vi "模拟输入_连续(IEPE_频域).vi"() -> ()   [LabVIEW 2013]
doc: "This example demonstrates how to acquire a continuous data."
uses:
  <userlib>/ArtDAQ/_SubVI/ArtDAQ_CreateAIVoltageIEPEChan.vi
  <userlib>/ArtDAQ/_SubVI/ArtDAQ_CfgSampClkTiming.vi
  <userlib>/ArtDAQ/_SubVI/ArtDAQ_CfgDigEdgeStartTrig.vi
  <userlib>/ArtDAQ/_SubVI/ArtDAQ_CfgAnlgEdgeStartTrig.vi
  <userlib>/ArtDAQ/_SubVI/ArtDAQ_Read Analog DBL NChan NSamp.vi
  <vilib>/measure/maspectr.llb/FFT Power Spectrum and PSD for 1 Chan.vi
  <vilib>/measure/NI_MAPro.lvlib
panel:
  out "波形图":cluster{"f0":dbl, "df":dbl, "magnitude":dbl[]}[](graph)
  in  "耦合":i32(ring)=10050 items=["交流耦合"=10045, "直流耦合"=10050, "接地"=10066]
  in  "触发模式":enum32{"无触发", "数字边沿", "模拟边沿"}(tab)
  in  "触发源":string="/Dev1/PFI1"
  in  "触发边沿":i32(ring)=10280 items=["上升"=10280, "下降"=10171]
  in  "触发电平(V)":dbl
  in  "触发源":string(combo)="Dev1/ai0"
  in  "斜率":i32(ring)=10280 items=["上升"=10280, "下降"=10171]
  in  "停止":bool
  out "波形图":dbl[][](graph)
  in  "采样速率":dbl=10000.0 format="%#_13g"
  in  "每通道采样数":i32=1000
  in  "接线端配置":i32(ring)=12529 items=["默认"=-1, "单端"=10083, "非参考单端"=10078, "差分"=10106, "伪差分"=12529]
  in  "最小值(V)":dbl=-11.0 format="%#_13g"
  in  "最大值(V)":dbl=11.0 format="%#_13g"
  in  "物理通道":string(combo)="Dev1/ai0"
  out "错误":errorcluster
  # "通道属性"
  # "定时"
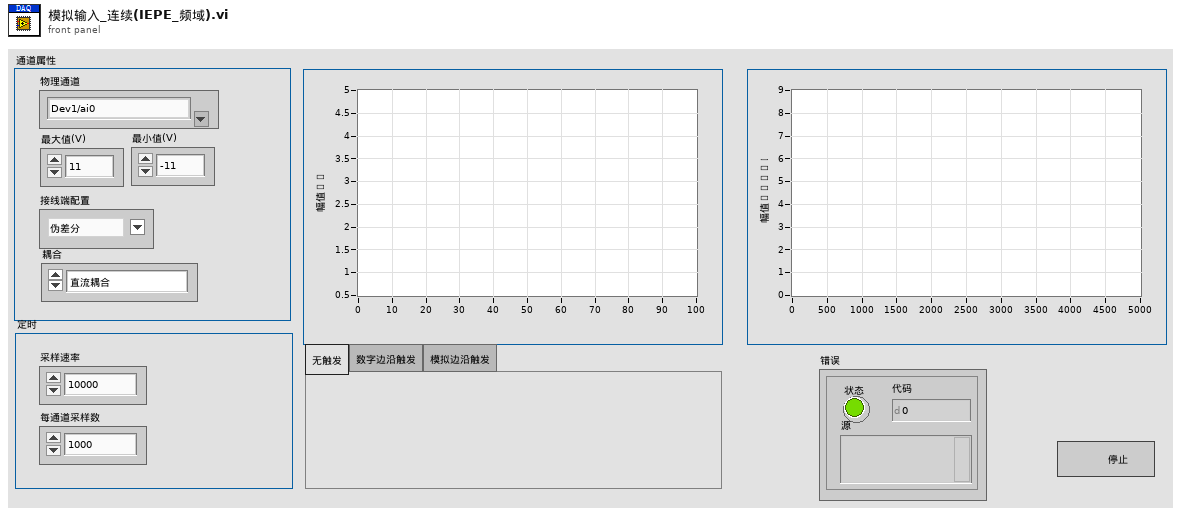
[diagram p1: front panel]
types:
  T1 = cluster{"averaging mode":enum16{"No averaging", "Vector averaging", "RMS averaging", "Peak hold"}, "weighting mode":enum16{"Linear", "Exponential"}, "number of averages":u32}
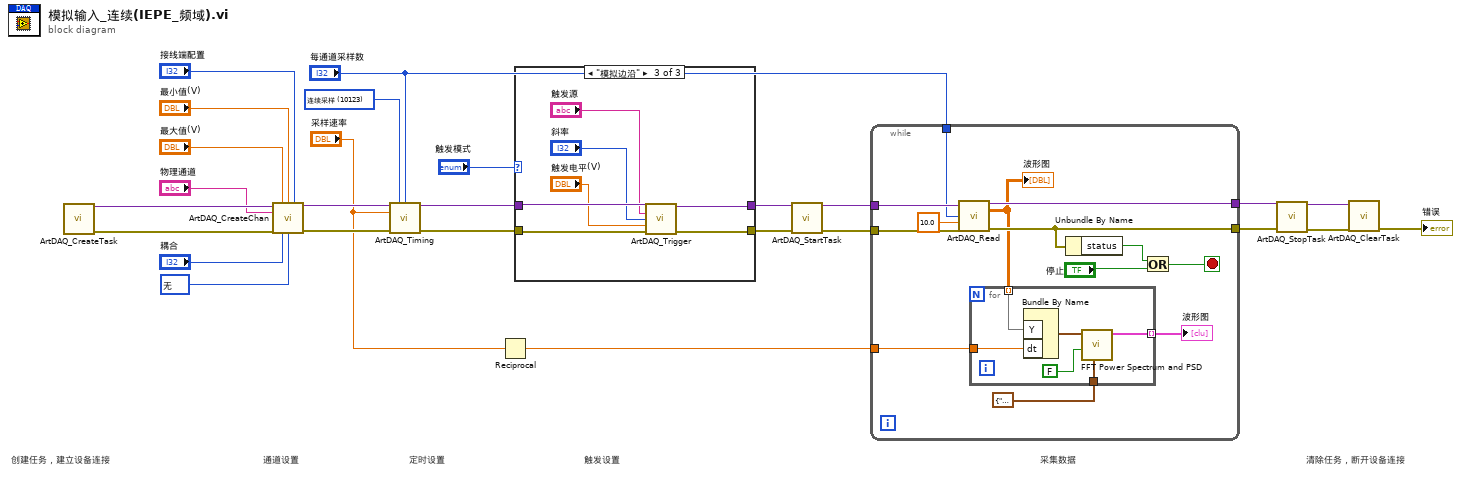
[diagram p0: block diagram]
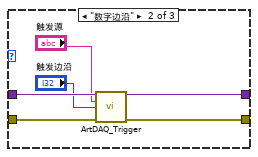
[diagram p3: hidden frame]
diagram:
  w3 = 10230 items=["内部"=10200, "外部"=10167, "无"=10230] ("电流激励源")
  w21 = 10123 items=["有限点采样"=10178, "连续采样"=10123] ("SampleMode")
  # "清除任务，断开设备连接"
  # "采集数据"
  # "触发设置"
  # "定时设置"
  # "通道设置"
  # "创建任务，建立设备连接"
  n1 = call <userlib>:"ArtDAQ_CreateTask.vi"() -> ("任务句柄"=w16:variant, "错误输出"=w26:errorcluster)  [unwired: 14 in]
  n2 = call-poly <userlib>:"ArtDAQ_CreateChan.vi"("任务句柄"=w16, "最大值"="最大值(V)", "最小值"="最小值(V)", "接线端配置"="接线端配置", "物理通道"="物理通道", "错误输入"=w26, "耦合方式"="耦合", "电流激励源"=w3) -> ("任务句柄"=w5:variant, "错误输出"=w22:errorcluster)  [unwired: 6 in]
  n3 = call-poly <userlib>:"ArtDAQ_Timing.vi"("任务句柄"=w5, "采样模式"=w21, "每通道采样数"="每通道采样数", "采样率"="采样速率", "错误输入"=w22) -> ("任务句柄"=w10:variant, "错误输出"=w8:errorcluster)  [unwired: 9 in]
  n4 = Reciprocal(x="采样速率") -> (1/x=w1:dbl)
  n5 = case shown="\"模拟边沿\"" "触发模式" {
    tunnel: w10 -> [w28 w34 w41]
    tunnel: [w28 w33 w40] -> w9
    tunnel: w8 -> [w27 w31 w38]
    tunnel: [w27 w32 w39] -> w7
    frame "无触发", Default {
    }
    frame "数字边沿" {
      n6 = call-poly <userlib>:"ArtDAQ_Trigger.vi"("任务句柄"=w34, "触发源"="触发源", "边沿"="触发边沿", "错误输入"=w31) -> ("任务句柄"=w33:variant, "错误输出"=w32:errorcluster)  [unwired: 10 in]
    }
    frame "模拟边沿" {
      n7 = call-poly <userlib>:"ArtDAQ_Trigger.vi"("任务句柄"=w41, "触发源"="触发源", "斜率"="斜率", "触发电平"="触发电平(V)", "错误输入"=w38) -> ("任务句柄"=w40:variant, "错误输出"=w39:errorcluster)  [unwired: 9 in]
    }
  }
  n8 = call <userlib>:"ArtDAQ_StartTask.vi"("任务句柄"=w9, "错误输入"=w7) -> ("任务句柄"=w19:variant, "错误输出"=w18:errorcluster)  [unwired: 12 in]
  n9 = while {
    tunnel: w19 -> [w54]
    tunnel: w18 -> [w53]
    tunnel: "每通道采样数" -> [w52]
    tunnel: [w50] -> w15
    tunnel: [w49] -> w14
    tunnel: w1 -> [w44]
    stop <- w47 stop-if-true
    n10 = call-poly <userlib>:"ArtDAQ_Read.vi"("任务句柄"=w54, "每通道采样数"=w52, "超时s"=10.0 ("Timeout"), "错误输入"=w53) -> ("任务句柄"=w50:variant, "数据"=w45:dbl[][], "错误输出"=w49:errorcluster)  [unwired: 8 in, 1 out]
    "波形图" <- w45
    n11 = for {
      tunnel: w45 -> [w59] mode=indexing
      tunnel: w44 -> [w58]
      tunnel: [w57] -> w43 mode=indexing
      tunnel: T1 {"averaging mode"=enum."No averaging", "weighting mode"=enum."Linear", "number of averages"=10} ("averaging parameters") -> [w56]
      n12 = Bundle By Name("Y"=w59, "dt"=w58) -> (w60:waveform(dbl))  [unwired: 1 in]
      n13 = call-poly <vilib>:"FFT Power Spectrum and PSD.vi"("averaging parameters"=w56, "dB On (F)"=FALSE, "time signal"=w60) -> ("Power Spectrum / PSD"=w57:cluster{"f0":dbl, "df":dbl, "magnitude":dbl[]})  [unwired: 5 in, 3 out]
    }
    "波形图" <- w43
    n14 = Unbundle By Name(w49) -> ("status"=w48:bool)
    n15 = Or(x=w48, y="停止") -> (x .or. y?=w47:bool)
  }
  n16 = call <userlib>:"ArtDAQ_StopTask.vi"("任务句柄"=w15, "错误输入"=w14) -> ("任务句柄"=w13:variant, "错误输出"=w12:errorcluster)  [unwired: 12 in]
  n17 = call <userlib>:"ArtDAQ_ClearTask.vi"("任务句柄"=w13, "错误输入"=w12) -> ("错误输出"=→"错误":errorcluster)  [unwired: 13 in]
